vi "Set Time.vi"(6 "Remote Timeout (300,000 ms)":u32=300000, 8 "error in (no error)":errorcluster, 9 "Time Zone":string, 10 "Time":timestamp, 11 "Session in (localhost)":refnum<k21>="localhost") -> (0 "error out":errorcluster, 1 "Changes Require Restart":bool, 2 "Detailed Result":string, 3 "Session out":refnum<k21>)   [LabVIEW 2014, in "nisyscfg.lvlib"]
doc: "Sets the current time and/or time zone on the specified system."
uses:
  nisyscfg.lvlib
  Save Changes (Hardware).vi
  Close (Hardware).vi
  C:/Program Files (x86)/National Instruments/LabVIEW 2014/resource/objmgr/nisysapi.rc
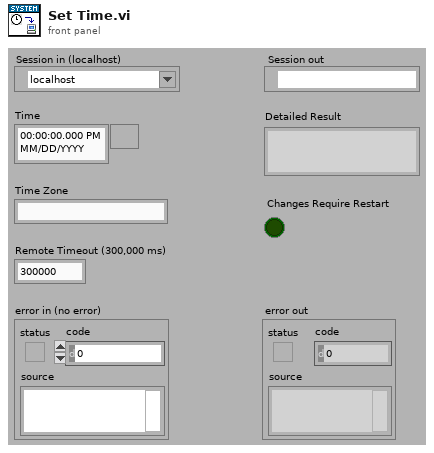
[diagram p1: front panel]
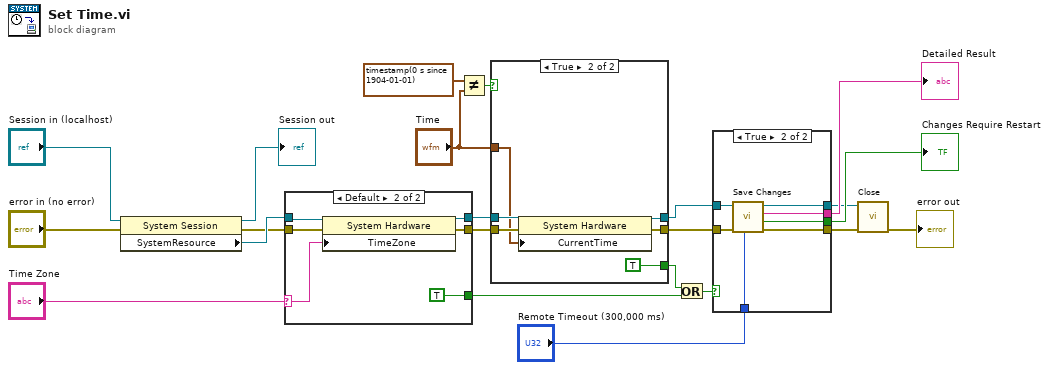
[diagram p0: block diagram]
diagram:
  n1 = property class="System Session"(reference="Session in (localhost)", error in="error in (no error)") -> (reference out=→"Session out":refnum<k21>, error out=w15:errorcluster, "SystemResource"=w18:refnum<k20>)
  n2 = case shown="Default" "Time Zone" {
    selector: "Time Zone" -> [_ w26]
    tunnel: w18 -> [w24 w30]
    tunnel: w15 -> [w23 w29]
    tunnel: [w23 w28] -> w11
    tunnel: [w24 w27] -> w10
    tunnel: [_ TRUE] -> w2
    frame "" {
    }
    frame Default {
      n3 = property class="System Hardware"(reference=w30, error in=w29, "TimeZone"=w26) -> (reference out=w27:refnum<k20>, error out=w28:errorcluster)
    }
  }
  n4 = Not Equal?(x=timestamp(0 s since 1904-01-01) ("Time"), y="Time") -> (x != y?=w6:bool)
  n5 = case shown="True" w6 {
    tunnel: w11 -> [w31 w38]
    tunnel: w10 -> [w32 w37]
    tunnel: "Time" -> [_ w36]
    tunnel: [w32 w35] -> w9
    tunnel: [w31 w34] -> w8
    tunnel: [_ TRUE] -> w3
    frame False {
    }
    frame True {
      n6 = property class="System Hardware"(reference=w37, error in=w38, "CurrentTime"=w36) -> (reference out=w35:refnum<k20>, error out=w34:errorcluster)
    }
  }
  n7 = Or(x=w3, y=w2) -> (x .or. y?=w1:bool)
  n8 = case shown="True" w1 {
    tunnel: [w40 w47] -> w13
    tunnel: [w39 w46] -> w12
    tunnel: w9 -> [w40 w45]
    tunnel: w8 -> [w39 w44]
    tunnel: [_ w43] -> w22
    tunnel: [_ w42] -> w20
    tunnel: "Remote Timeout (300,000 ms)" -> [_ w41]
    frame False {
    }
    frame True {
      n9 = call-poly "Save Changes.vi"("Remote Timeout (300,000 ms)"=w41, "error in (no error)"=w44, "Resource in"=w45) -> ("error out"=w46:errorcluster, "Changes Require Restart"=w43:bool, "Detailed Result"=w42:string, "Resource out"=w47:refnum<k20>)  [unwired: 5 in]
    }
  }
  "Changes Require Restart" <- w22
  "Detailed Result" <- w20
  n10 = call-poly "Close.vi"("error in (no error)"=w12, "Resource in"=w13) -> ("error out"=→"error out":errorcluster)  [unwired: 9 in]
